vi "Draw Speaker.vi"(0 "picture in":picture, 5 "center":cluster{"X":i32, "Y":i32}, 7 "width":i32, 9 "state":T1, 11 "active":bool) -> (4 "picture out":picture)   [LabVIEW 2015, in "HRTF Config.xctl"]
uses:
  HRTF Config.xctl
  Speaker State.ctl
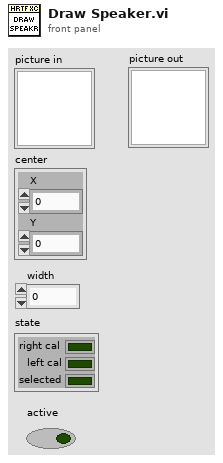
[diagram p1: front panel]
types:
  T1 = typedef "HRTF Config.xctl/Speaker State.ctl" = cluster{"right cal":bool, "left cal":bool, "selected":bool}
  T2 = cluster{"Width":u16, "Style":enum32{"Solid", "Dash", "Dot", "DashDot", "DashDotDot"}}
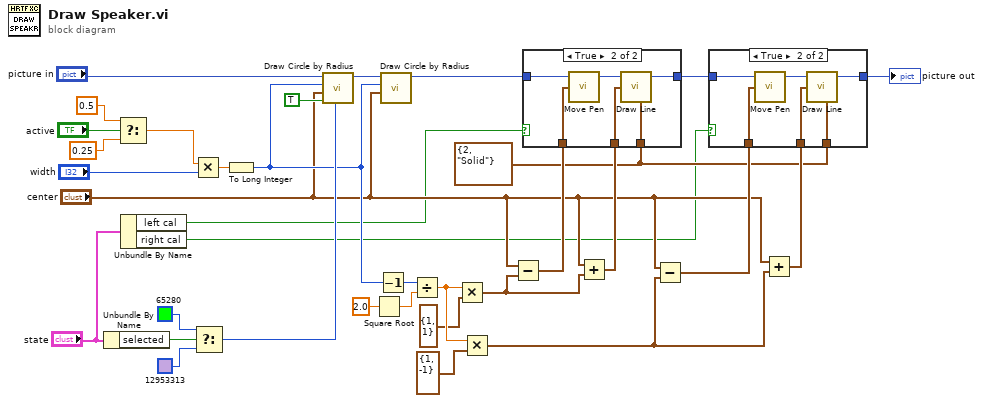
[diagram p0: block diagram]
diagram:
  w4 = T2 {"Width"=2, "Style"=enum."Solid"} ("pen")
  n1 = Unbundle By Name("state") -> ("selected"=w25:bool)
  n2 = Select(t=0.5, s="active", f=0.25) -> (s? t:f=w27:dbl)
  n3 = Unbundle By Name("state") -> ("left cal"=w2:bool, "right cal"=w1:bool)
  n4 = Multiply(x=w27, y="width") -> (x*y=w30:dbl)
  n5 = Select(t=u32 65280 ("color(black)"), s=w25, f=u32 12953313 ("color(black)")) -> (s? t:f=w22:u32)
  n6 = To Long Integer(number=w30) -> (32bit integer=w21:i32)
  n7 = call <vilib>:"Draw Circle by Radius.vi"("color(black)"=w22, "fill?(F)"=TRUE, "pixel center"="center", "radius"=w21, "picture"="picture in") -> ("new picture"=w34:picture)  [unwired: 6 in]
  n8 = Square Root(x=2.0) -> (sqrt(x)=w19:dbl)
  n9 = Decrement(x=w21) -> (x-1=w20:i32)
  n10 = call <vilib>:"Draw Circle by Radius.vi"("pixel center"="center", "radius"=w21, "picture"=w34) -> ("new picture"=w17:picture)  [unwired: 8 in]
  n11 = Divide(x=w20, y=w19) -> (x/y=w15:dbl)
  n12 = Multiply(x=w15, y=cluster{"x":i16, "y":i16} {"x"=1, "y"=1} ("new position")) -> (x*y=w12:cluster{"x":dbl, "y":dbl})
  n13 = Multiply(x=w15, y=cluster{"x":i16, "y":i16} {"x"=1, "y"=-1} ("new position")) -> (x*y=w7:cluster{"x":dbl, "y":dbl})
  n14 = Subtract(x="center", y=w12) -> (x-y=w13:cluster{dbl, dbl})
  n15 = Add(x="center", y=w12) -> (x+y=w11:cluster{dbl, dbl})
  n16 = case shown="True" w2 {
    tunnel: w17 -> [w35 w41]
    tunnel: w13 -> [_ w40]
    tunnel: w11 -> [_ w38]
    tunnel: [w35 w37] -> w10
    tunnel: w4 -> [_ w36]
    frame False {
    }
    frame True {
      n17 = call <vilib>:"Move Pen.vi"("new position"=w40, "picture"=w41) -> ("new picture"=w39:picture)  [unwired: 3 in]
      n18 = call <vilib>:"Draw Line.vi"("picture"=w39, "end point"=w38, "pen"=w36) -> ("new picture"=w37:picture)  [unwired: 6 in]
    }
  }
  n19 = Subtract(x="center", y=w7) -> (x-y=w9:cluster{dbl, dbl})
  n20 = Add(x="center", y=w7) -> (x+y=w6:cluster{dbl, dbl})
  n21 = case shown="True" w1 {
    tunnel: w10 -> [w42 w48]
    tunnel: w9 -> [_ w47]
    tunnel: w6 -> [_ w45]
    tunnel: [w42 w44] -> w5
    tunnel: w4 -> [_ w43]
    frame False {
    }
    frame True {
      n22 = call <vilib>:"Move Pen.vi"("new position"=w47, "picture"=w48) -> ("new picture"=w46:picture)  [unwired: 3 in]
      n23 = call <vilib>:"Draw Line.vi"("picture"=w46, "end point"=w45, "pen"=w43) -> ("new picture"=w44:picture)  [unwired: 6 in]
    }
  }
  "picture out" <- w5
